vi "CANcoderGetters.vi"   [LabVIEW 2023]
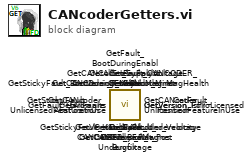
[diagram p0: block diagram]
diagram:
  n1 = call <vilib>:"GetStickyFault_CANCODER_BadMagnet.vi"() -> ()  [unwired: 11 in, 1 out]
  n2 = call <vilib>:"GetFault_CANCODER_BadMagnet.vi"() -> ()  [unwired: 11 in, 1 out]
  n3 = call <vilib>:"GetStickyFault_UnlicensedFeatureInUse.vi"() -> ()  [unwired: 11 in, 1 out]
  n4 = call <vilib>:"GetFault_UnlicensedFeatureInUse.vi"() -> ()  [unwired: 11 in, 1 out]
  n5 = call <vilib>:"GetStickyFault_BootDuringEnable.vi"() -> ()  [unwired: 11 in, 1 out]
  n6 = call <vilib>:"GetFault_BootDuringEnable.vi"() -> ()  [unwired: 11 in, 1 out]
  n7 = call <vilib>:"GetStickyFault_Undervoltage.vi"() -> ()  [unwired: 11 in, 1 out]
  n8 = call <vilib>:"GetFault_Undervoltage.vi"() -> ()  [unwired: 11 in, 1 out]
  n9 = call <vilib>:"GetStickyFault_Hardware.vi"() -> ()  [unwired: 11 in, 1 out]
  n10 = call <vilib>:"GetFault_Hardware.vi"() -> ()  [unwired: 11 in, 1 out]
  n11 = call <vilib>:"GetVersion_IsProLicensed.vi"() -> ()  [unwired: 11 in, 1 out]
  n12 = call <vilib>:"GetCANcoder_MagHealth.vi"() -> ()  [unwired: 11 in, 1 out]
  n13 = call <vilib>:"GetCANCoder_SupplyVoltage.vi"() -> ()  [unwired: 11 in, 1 out]
  n14 = call <vilib>:"GetCANCoder_RawPos.vi"() -> ()  [unwired: 11 in, 1 out]
  n15 = call <vilib>:"GetCANCoder_RawVel.vi"() -> ()  [unwired: 11 in, 1 out]
  n16 = call <vilib>:"GetCANcoder_AbsPosition.vi"() -> ()  [unwired: 11 in, 1 out]
  n17 = call <vilib>:"GetCANcoder_Position.vi"() -> ()  [unwired: 11 in, 1 out]
  n18 = call <vilib>:"GetCANcoder_Velocity.vi"() -> ()  [unwired: 11 in, 1 out]
  n19 = call <vilib>:"GetAllStickyFaults.vi"() -> ()  [unwired: 11 in, 1 out]
  n20 = call <vilib>:"GetAllFaults.vi"() -> ()  [unwired: 11 in, 1 out]
  n21 = call <vilib>:"GetVersion_Full.vi"() -> ()  [unwired: 11 in, 1 out]
  n22 = call <vilib>:"GetVersion_Build.vi"() -> ()  [unwired: 11 in, 1 out]
  n23 = call <vilib>:"GetVersion_Bugfix.vi"() -> ()  [unwired: 11 in, 1 out]
  n24 = call <vilib>:"GetVersion_Minor.vi"() -> ()  [unwired: 11 in, 1 out]
  n25 = call <vilib>:"GetVersion_Major.vi"() -> ()  [unwired: 11 in, 1 out]
